vi "write Port.vi"(8 "error in (no error)":errorcluster, 9 "length":i32, 10 "packet":string, 11 "port_num":i32) -> (0 "error out":errorcluster, 2 "packet out":string, 3 "function return":i32)   [LabVIEW 2022 SP3, in "dxl.lvlib"]
doc: "WINDECLSPEC int writePort (int port_num, uint8_t *packet, int length);"
uses:
  dxl.lvlib
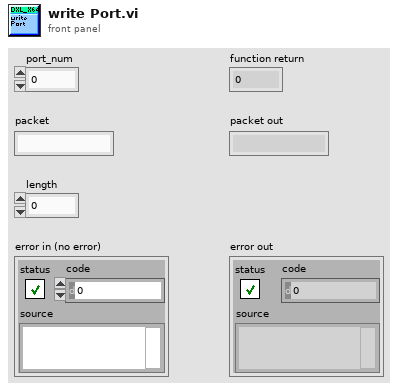
[diagram p1: front panel]
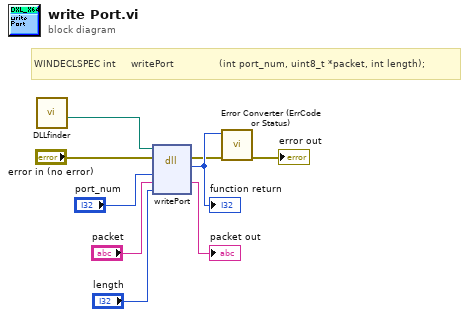
[diagram p0: block diagram]
diagram:
  # "WINDECLSPEC int     writePort               (int port_num, uint8_t *packet, int length);"
  n1 = call "DLLfinder.vi"() -> ("File Path"=w1:path)  [unwired: 11 in]
  n2 = dll-call lib="C:/EnFlo_Software/ADAM Serial/Instrument drivers/Dynamixel/2nd attempt/Library/dxl_x64_c.*" fn="writePort"(path in=w1, error in="error in (no error)", "port_num"="port_num", "packet"="packet", "length"="length") -> (error out=w3:errorcluster, "return type"=w9:i32, "packet"=→"packet out":string)  [unwired: 3 in, 1 out]
  "function return" <- w9
  n3 = call "Error Converter (ErrCode or Status).vi"("error in (no error)"=w3, "error code"=w9) -> ("error out"=→"error out":errorcluster)  [unwired: 9 in]
